vi "Run Test (VIRefnum Scalar).vi"(5 "Test Report":refnum<class "Test Report.lvclass">, 6 "Verbose":bool, 7 "Report Path":path, 8 "error in":errorcluster, 9 "Inspect Recursively (T)":bool=TRUE, 10 "VI Refnum":refnum<vi>, 11 "Interactive (T)":bool=TRUE) -> (0 "error out":errorcluster)   [LabVIEW 2013, in "Caraya.lvlib"]
uses:
  classes/Test Report/Test Report.lvclass
  Caraya.lvlib
  classes/Test Runner/Test Runner.lvclass
  classes/Test Runner.Folder/Test Runner.Folder.lvclass
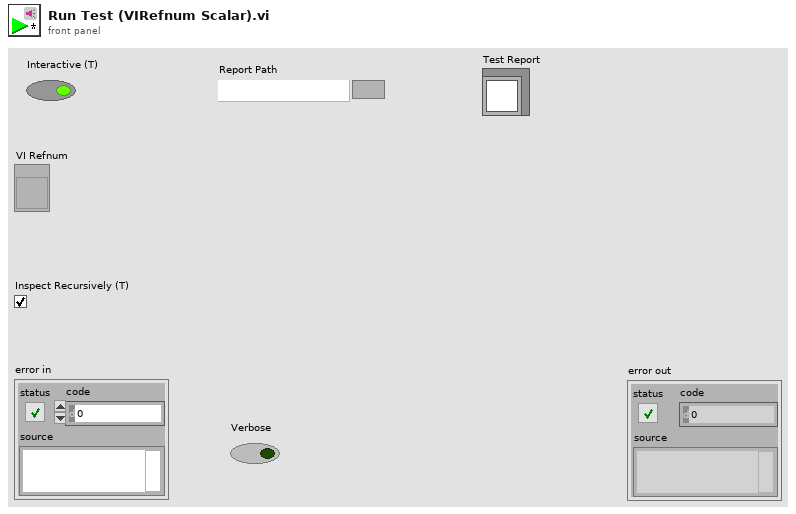
[diagram p1: front panel]
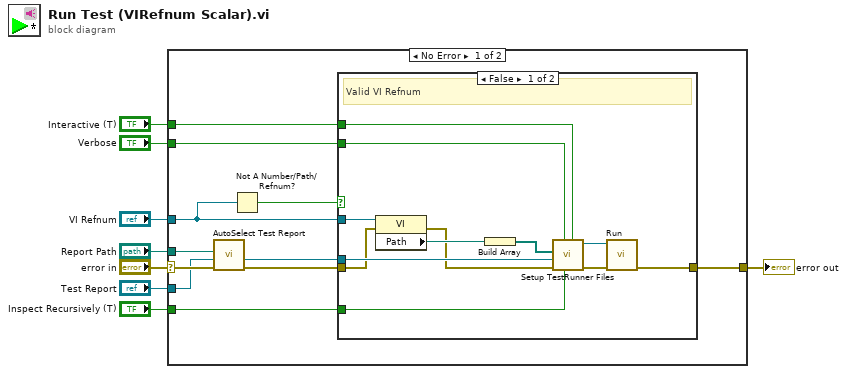
[diagram p0: block diagram]
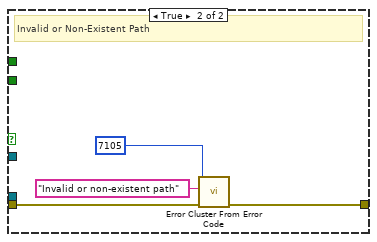
[diagram p2: hidden frame]
diagram:
  n1 = case shown="No Error" "error in" {
    selector: "error in" -> [w16 w36]
    tunnel: [w19 w36] -> w8
    tunnel: "Verbose" -> [w18 _]
    tunnel: "Interactive (T)" -> [w17 _]
    tunnel: "Test Report" -> [w13 _]
    tunnel: "VI Refnum" -> [w10 _]
    tunnel: "Report Path" -> [w15 _]
    tunnel: "Inspect Recursively (T)" -> [w11 _]
    frame No Error {
      n2 = call "AutoSelect Test Report.vi"("error in (no error)"=w16, "Test Report in"=w13, "Report Path"=w15) -> ("error out"=w14:errorcluster, "Test Report out"=w12:refnum<class "Test Report.lvclass">)  [unwired: 7 in]
      n3 = Not A Number/Path/Refnum?(number/path/refnum=w10) -> (NaN/Path/Refnum?=w9:bool)
      n4 = case shown="False" w9 {
        tunnel: [w31 w34] -> w19
        tunnel: w18 -> [w29 _]
        tunnel: w17 -> [w28 _]
        tunnel: w14 -> [w21 w35]
        tunnel: w12 -> [w26 _]
        tunnel: w11 -> [w25 _]
        tunnel: w10 -> [w23 _]
        frame False {
          # "Valid VI Refnum"
          n5 = property class="VI"(reference=w23, error in=w21) -> (error out=w20:errorcluster, "Path"=w22:path)  [unwired: 1 out]
          n6 = Build Array(w22) -> (w24:path[])
          n7 = call "Setup TestRunner Files.vi"("Interactive (T)"=w28, "Inspect Recursively (T)"=w25, "Verbose (F)"=w29, "error in (no error)"=w20, "Test Report"=w26, "Paths"=w24) -> ("error out"=w30:errorcluster, "Test Runner.Folder out"=w27:refnum<class "Test Runner.Folder.lvclass">)  [unwired: 4 in]
          n8 = call "Run.vi"("error in (no error)"=w30, "Test Runner in"=w27) -> ("error out"=w31:errorcluster)  [unwired: 8 in, 1 out]
        }
        frame True {
          # "Invalid or Non-Existent Path"
          n9 = call <vilib>:"Error Cluster From Error Code.vi"("error in (no error)"=w35, "error message (\"\")"="Invalid or non-existent path" ("error message (\"\")"), "error code (0)"=7105 ("code")) -> ("error out"=w34:errorcluster)  [unwired: 6 in]
        }
      }
    }
    frame Error {
    }
  }
  "error out" <- w8
